vi "Run.vi"(8 "error in (no error)":errorcluster, 11 "API":T1) -> (0 "error out":errorcluster, 3 "API dup":T1)   [LabVIEW 2013, in "SMOFacade.lvclass"]
uses:
  SMOFacade.lvclass
  Registry/SMO_API--Cluster.ctl
  Terminal/SMOTerminal.lvclass
  Registry/Registry-SMO.lvclass
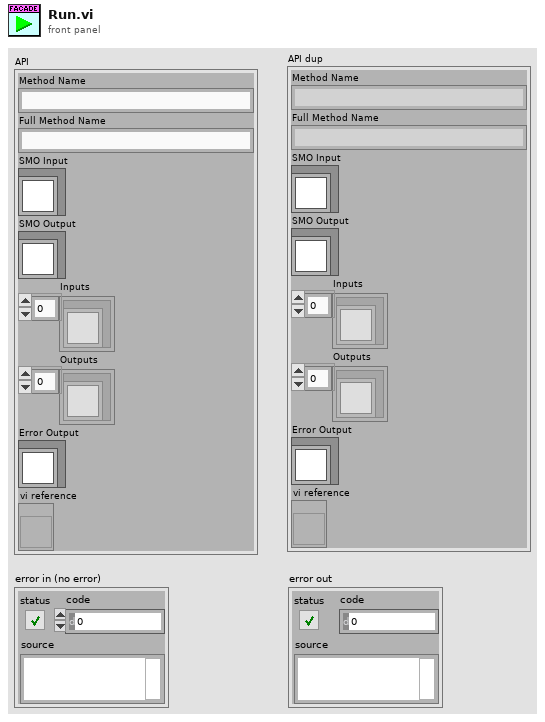
[diagram p1: front panel]
types:
  T1 = typedef "Registry-SMO.lvclass/SMO_API--Cluster.ctl" = cluster{"Method Name":string, "Full Method Name":string, "SMO Input":refnum<class "SMOTerminal.lvclass">, "SMO Output":refnum<class "SMOTerminal.lvclass">, "Inputs":refnum<class "SMOTerminal.lvclass">[], "Outputs":refnum<class "SMOTerminal.lvclass">[], "Error Output":refnum<class "SMOTerminal.lvclass">, "vi reference":refnum<vi>}
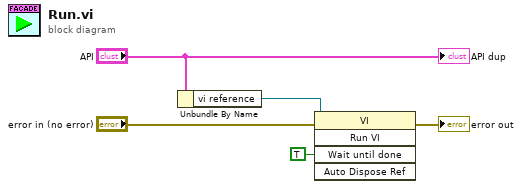
[diagram p0: block diagram]
diagram:
  n1 = Unbundle By Name("API") -> ("vi reference"=w2:refnum<vi>)
  n2 = invoke class="VI" method="Run VI"(reference=w2, error in="error in (no error)", "Wait until done"=TRUE ("Wait Until Done")) -> (error out=→"error out":errorcluster)  [unwired: 2 in, 4 out]
  "API dup" <- "API"
